vi "2 XYPointsToDistanceAndAngle.vi"(8 "East 2":dbl, 9 "North 2":dbl, 10 "East 1":dbl, 11 "North 1":dbl) -> (2 "Angle Diff":dbl, 3 "Distance":dbl)   [LabVIEW 2011]
doc: "given two points in cartesian coordinates, this VI outputs the distance between them and the angle from the vertical to the line connecting the two points"
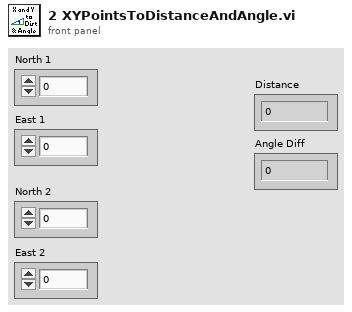
[diagram p1: front panel]
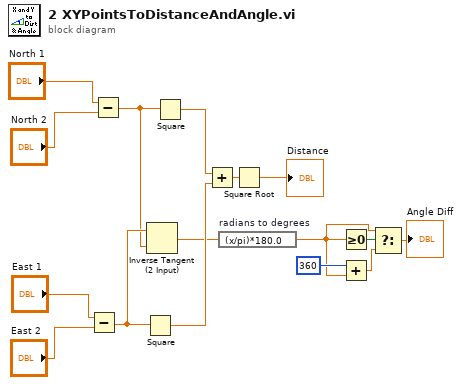
[diagram p0: block diagram]
diagram:
  n1 = Subtract(x="East 1", y="East 2") -> (x-y=w8:dbl)
  n2 = Subtract(x="North 1", y="North 2") -> (x-y=w7:dbl)
  n3 = Square(x=w8) -> (x^2=w11:dbl)
  n4 = Inverse Tangent (2 Input)(1:w7, 2:w8) -> (0:w1:dbl)
  n5 = Square(x=w7) -> (x^2=w12:dbl)
  n6 = Add(x=w12, y=w11) -> (x+y=w10:dbl)
  n7 = expression code="(x/pi)*180.0" "radians to degrees"(w1) -> (w2:dbl)
  n8 = Square Root(x=w10) -> (sqrt(x)=→"Distance":dbl)
  n9 = Greater Or Equal To 0?(x=w2) -> (x >= 0?=w5:bool)
  n10 = Add(x=360, y=w2) -> (x+y=w3:dbl)
  n11 = Select(t=w2, s=w5, f=w3) -> (s? t:f=→"Angle Diff":dbl)
